vi "Copy Graph Attributes.vi"(8 "error in (no error)":errorcluster, 10 "Copy to":refnum<vi>, 11 "Copy from":refnum<vi>) -> (0 "error out":errorcluster)   [LabVIEW 2016]
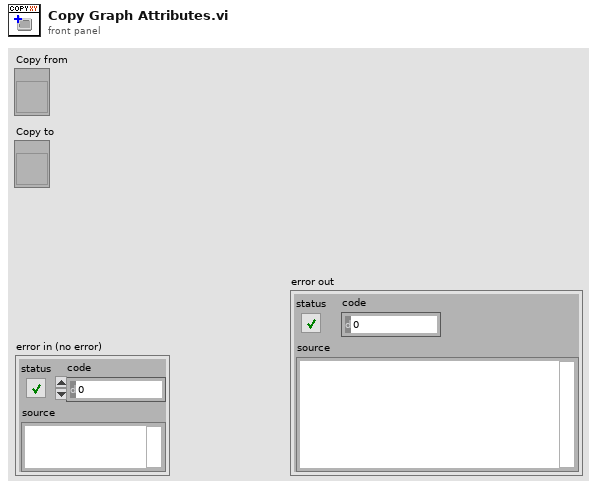
[diagram p1: front panel]
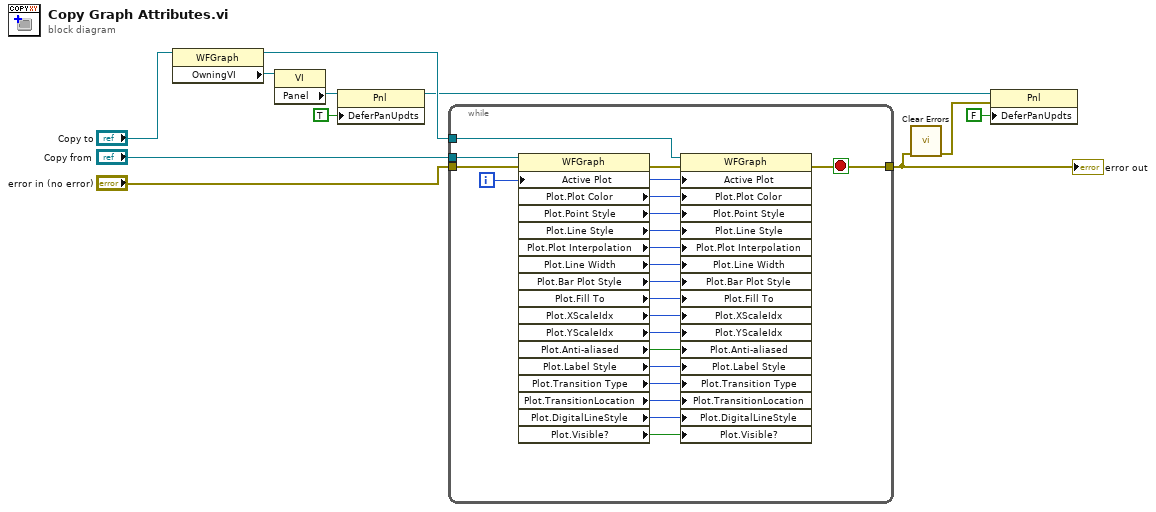
[diagram p0: block diagram]
diagram:
  n1 = property class="WFGraph"(reference="Copy to") -> (reference out=w6:refnum<vi>, "OwningVI"=w9:refnum<vi>)  [unwired: 1 in, 1 out]
  n2 = property class="VI"(reference=w9) -> ("Panel"=w8:refnum<vi>)  [unwired: 1 in, 2 out]
  n3 = property class="Pnl"(reference=w8, "DeferPanUpdts"=TRUE ("Defer Panel Updates")) -> (reference out=w2:refnum<vi>)  [unwired: 1 in, 1 out]
  n4 = while {
    tunnel: "Copy from" -> [w32]
    tunnel: w6 -> [w30]
    tunnel: "error in (no error)" -> [w31]
    tunnel: [w28] -> w4
    i -> [w27]
    stop <- w28 stop-if-true
    n5 = property class="WFGraph"(reference=w32, error in=w31, "Active Plot"=w27) -> (error out=w29:errorcluster, "Plot.Plot Color"=w26:u32, "Plot.Point Style"=w25:u8, "Plot.Line Style"=w24:u8, "Plot.Plot Interpolation"=w23:u8, "Plot.Line Width"=w22:u8, "Plot.Bar Plot Style"=w21:u8, "Plot.Fill To"=w20:i16, "Plot.XScaleIdx"=w19:u32, "Plot.YScaleIdx"=w18:u32, "Plot.Anti-aliased"=w17:bool, "Plot.Label Style"=w16:u8, "Plot.Transition Type"=w15:u8, "Plot.TransitionLocation"=w14:u8, "Plot.DigitalLineStyle"=w13:u8, "Plot.Visible?"=w12:bool)  [unwired: 1 out]
    n6 = property class="WFGraph"(reference=w30, error in=w29, "Active Plot"=w27, "Plot.Plot Color"=w26, "Plot.Point Style"=w25, "Plot.Line Style"=w24, "Plot.Plot Interpolation"=w23, "Plot.Line Width"=w22, "Plot.Bar Plot Style"=w21, "Plot.Fill To"=w20, "Plot.XScaleIdx"=w19, "Plot.YScaleIdx"=w18, "Plot.Anti-aliased"=w17, "Plot.Label Style"=w16, "Plot.Transition Type"=w15, "Plot.TransitionLocation"=w14, "Plot.DigitalLineStyle"=w13, "Plot.Visible?"=w12) -> (error out=w28:errorcluster)  [unwired: 1 out]
  }
  "error out" <- w4
  n7 = call <vilib>:"Clear Errors.vi"("error in (no error)"=w4) -> ("error out"=w3:errorcluster)  [unwired: 5 in, 1 out]
  n8 = property class="Pnl"(reference=w2, error in=w3, "DeferPanUpdts"=FALSE ("Defer Panel Updates")) -> ()  [unwired: 2 out]
